vi "Launch DS Server if Local URL.vi"(4 "error in (no error)":errorcluster, 7 "URL":string) -> (0 "error out":errorcluster, 3 "Duplicate URL":string)   [LabVIEW 2018]
doc: "If the URL input refers to the DataSocket server on this machine (for example \"dstp://localhost/wave\"), then the DataSocket server is started."
panel:
  in  "type specifier VI Refnum (for type only)":refnum<vi>
  in  "Message":string="Launching the DataSocket Server is currently not supported on non-windows platforms. Please try connecting to a DataSocket Server running on windows."
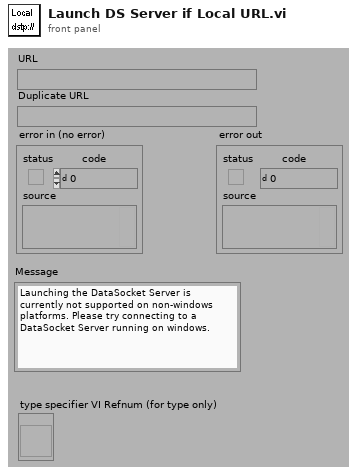
[diagram p1: front panel]
types:
  T1 = enum32{"invalid OS target", "Mac OS", "Windows 3.1", "Windows 95/NT", "Solaris 1", "Solaris 2", "HP-UX", "PowerMAX", "Linux", "Irix", "Rhapsody", "BeOS", "AIX", "OSF1", "VxWorks", "PharLap", "Carbon"}
  T2 = enum32{"invalid OS target", "Mac OS", "Windows 3.1", "Windows 95/NT", "Solaris 1", "Solaris 2", "HP-UX", "PowerMAX", "Linux", "Irix", "Rhapsody", "BeOS", "AIX", "OSF1", "VxWorks", "PharLap", "Carbon", "RTX", "Windows x64", "Linux x64", "Mac OS X x64"}
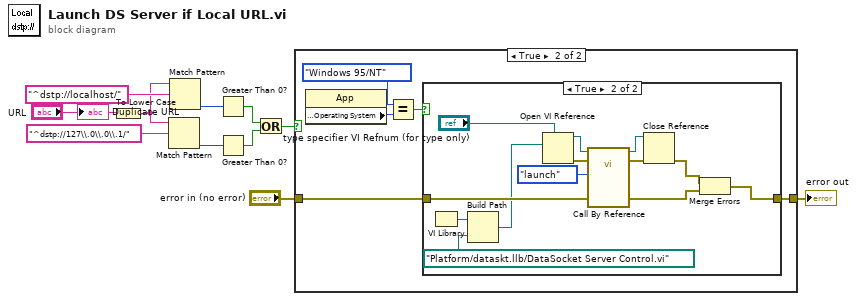
[diagram p0: block diagram]
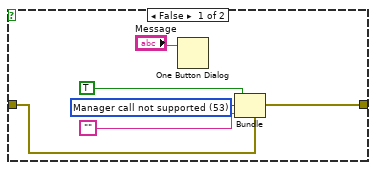
[diagram p3: hidden frame]
diagram:
  n1 = To Lower Case(string="URL") -> (all lower case string=w9:string)
  n2 = Match Pattern(string=w9, regular expression="^dstp://127\\.0\\.0\\.1/") -> (offset past match=w7:i32)  [unwired: 1 in, 3 out]
  n3 = Match Pattern(string=w9, regular expression="^dstp://localhost/") -> (offset past match=w8:i32)  [unwired: 1 in, 3 out]
  n4 = Greater Than 0?(x=w8) -> (x > 0?=w6:bool)
  n5 = Greater Than 0?(x=w7) -> (x > 0?=w5:bool)
  n6 = Or(x=w6, y=w5) -> (x .or. y?=w4:bool)
  n7 = case shown="True" w4 {
    tunnel: "error in (no error)" -> [w12 w14]
    tunnel: [w12 w17] -> w2
    frame False {
    }
    frame True {
      n8 = property class="App"() -> ("Application:Target:Operating System"=w15:T2)  [unwired: 2 in, 2 out]
      n9 = Equal?(x=T1."Windows 95/NT" ("Application:Target Operating System"), y=w15) -> (x = y?=w13:bool)
      n10 = case shown="True" w13 {
        tunnel: [w23 w30] -> w17
        tunnel: w14 -> [w18 w33]
        frame False {
          w19 = 53 items=["No error", "Argument error", "Memory is full", "Out of zone", "End of file", "File already open", "Generic file I/O error", "File not found", "File permission error", "Disk is full", "Duplicate path", "Too many files open", "System feature not enabled", "Resource file not found", "Cannot add resource", "Resource not found", "Image not found", "Image memory error", "Pen does not exist", "Config type invalid", "Config token not found", "Config parse error", "Config memory error", "Bad external code format", "Bad external code offset", "External code not present", "Null window", "Destroy window error", "Null menu", "Print aborted", "Bad print record", "Print driver error", "Windows error during printing", "Memory error during printing", "Print dialog error", "Generic print error", "Invalid device refnum", "Device not found", "Device parameter error", "Device unit error", "Cannot open device", "Device call aborted", "Generic error", "Cancelled by user", "Object ID too low", "Object ID too high", "Object not in heap", "Unknown heap", "Unknown object (invalid DefProc)", "Unknown object (DefProc not in table)", "Message out of range", "Invalid (null) method", "Unknown message", "Manager call not supported", "Bad address", "Network operation in progress", "Network operation timed out", "Connection is busy", "Network attribute not supported", "Network error", "Address in use", "System out of memory", "Connection aborted", "Connection refused", "Not connected", "Already connected", "Connection closed", "Initialization error (interapplication manager)", "Bad occurrence", "Wait on unbound occurrence handler", "Occurrence queue overflow", "Datalog type conflict", "Unused", "Unrecognized type (interapplication manager)", "Memory corrupt", "Failed to make temporary DLL", "Old CIN version", "Drag socket not found", "Failed to load drop-object", "Failed to register OLE object", "Failed to release OLE object", "Format specifier type mismatch", "Unknown format specifier", "Too few format specifiers", "Too many format specifiers", "Scan failed", "Newer CIN version", "Error converting to variant", "Runtime menu error", "Password tampered", "Variant attribute not found", "Incompatible variant data type", "Event data is not available", "Event Store is not present", "Occurrence is not found", "Event Queue is not created", "Event info is not available", "Refnum passed is NULL", "Error retrieving Class GUID", "Error retrieving CoClass GUID", "Error retrieving TypeLib GUID.", "Bad built application magic bytes.", "Specific driver is different from the specific driver associated with the Logical Name.", "There is no session opened to the class driver.", "Max Error", "MAX - Error with config objects", "MAX - Error loading configuration", "MAX - Group not supported"]
          n11 = One Button Dialog(message="Message") -> ()  [unwired: 1 in, 1 out]
          n12 = Bundle(cluster=w18, "status"=TRUE, "code"=w19, "source"="") -> (w23:errorcluster)
        }
        frame True {
          n13 = VI Library() -> (path=w27:path)
          n14 = Build Path(base path=w27, name or relative path=path "Platform/dataskt.llb/DataSocket Server Control.vi") -> (appended path=w25:path)
          n15 = Open VI Reference(type specifier VI Refnum (for type only)="type specifier VI Refnum (for type only)", vi path=w25) -> (vi reference=w35:refnum<vi>, error out=w34:errorcluster)  [unwired: 4 in]
          n16 = call-by-ref "?"(reference=w35, error in=w34, "error in (no error)"=w33, "operation (launch)"=enum16{"launch", "show", "hide", "close"}."launch") -> (reference out=w31:refnum<vi>, error out=w32:errorcluster, "error out"=w28:errorcluster)  [unwired: 5 in]
          n17 = Close Reference(reference=w31, error in (no error)=w32) -> (error out=w29:errorcluster)
          n18 = Merge Errors(w29, w28) -> (w30:errorcluster)
        }
      }
    }
  }
  "error out" <- w2
  "Duplicate URL" <- "URL"
